vi "Init UAV Marker Position.vi"(0 "GMAP Control ref":refnum<k24>, 5 "Overlay Ref":refnum<k24>, 7 "lat":dbl=-31.1105459 format="%#_13g", 9 "lng":dbl=150.8617687 format="%#_13g", 11 "error in (no error)":errorcluster) -> (15 "error out":errorcluster)   [LabVIEW 2014]
uses:
  C:/Robotic Systems/Products/AgFalcon/Software/Ground Station/Data/Mapping DLL/GMap.NET.WindowsForms.dll
  Data/Mapping DLL/GMap.NET.WindowsForms.dll
  Aircraft Information/Controls/Aircraft GPS Data.ctl
  Aircraft Information/Controls/GPS Fix Type.ctl
  System.Drawing
  C:/Robotic Systems/Products/AgFalcon/Software/Ground Station/Data/Mapping DLL/GMap.NET.Core.dll
  Data/Mapping DLL/GMap.NET.Core.dll
  Aircraft Information/Sub VI/Set Aircraft GPS.vi
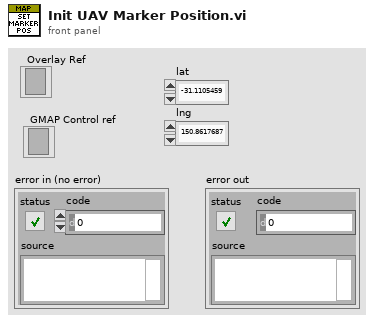
[diagram p1: front panel]
types:
  T1 = typedef "Aircraft GPS Data.ctl" = cluster{"Latitude (degrees)":dbl, "Longitude (degrees)":dbl, "Altitude (m)":dbl, "Fix Type":T2, "HDOP (cm)":u16, "VDOP (cm)":u16, "Ground Speed (m/s)":dbl, "Coarse Over Ground (degrees)":u16, "Number of Satellites":u8}
  T2 = typedef "GPS Fix Type.ctl" = enum16{"No Fix 0", "No Fix 1", "2D Fix", "3D Fix", "DGPS", "RTK"}
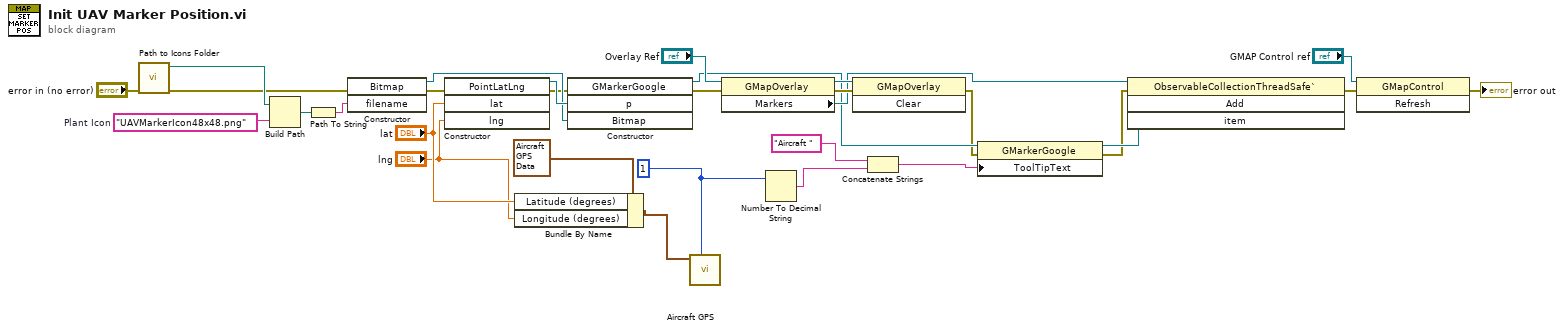
[diagram p0: block diagram]
diagram:
  w2 = u8 1 ("Aircraft ID")
  w18 = "UAVMarkerIcon48x48.png"  # Plant Icon
  n1 = call "Path to Icons Folder.vi"("Error In"="error in (no error)") -> ("Error Out"=w15:errorcluster, "Path to Icons Folder"=w19:path)  [unwired: 9 in]
  n2 = Build Path(base path=w19, name or relative path=w18) -> (appended path=w17:path)
  n3 = Path To String(path=w17) -> (string=w28:string)
  n4 = constructor class="Bitmap"(error in=w15, "filename"=w28) -> (reference out=w21:refnum<k24>, error out=w14:errorcluster)  [unwired: 2 in, 2 out]
  n5 = constructor class="PointLatLng"(error in=w14, "lat"="lat", "lng"="lng") -> (reference out=w27:refnum<k24>, error out=w13:errorcluster)  [unwired: 2 in, 3 out]
  n6 = Bundle By Name(cluster=T1 {"Latitude (degrees)"=0.0, "Longitude (degrees)"=0.0, "Altitude (m)"=0.0, "Fix Type"=enum."No Fix 0", "HDOP (cm)"=0, "VDOP (cm)"=0, "Ground Speed (m/s)"=0.0, "Coarse Over Ground (degrees)"=0, "Number of Satellites"=0} ("Aircraft Att Data Out"), "Latitude (degrees)"="lat", "Longitude (degrees)"="lng") -> (w1:T1)
  n7 = constructor class="GMarkerGoogle"(error in=w13, "p"=w27, "Bitmap"=w21) -> (reference out=w9:refnum<k24>, error out=w30:errorcluster)  [unwired: 2 in, 3 out]
  n8 = call-poly "Aircraft GPS.vi"("Aircraft ID"=w2, "Aircraft Att Data IN"=w1) -> ()  [unwired: 8 in, 2 out]
  n9 = property class="GMapOverlay"(reference="Overlay Ref", error in=w30) -> (reference out=w23:refnum<k24>, error out=w22:errorcluster, "Markers"=w20:refnum<k24>)
  n10 = Number To Decimal String(number=w2) -> (decimal integer string=w5:string)  [unwired: 1 in]
  n11 = invoke class="GMapOverlay" method="Clear"(reference=w23, error in=w22) -> (error out=w8:errorcluster)  [unwired: 1 in, 2 out]
  n12 = Concatenate Strings("Aircraft " ("string"), w5) -> (w3:string)
  n13 = property class="GMarkerGoogle"(reference=w9, error in=w8, "ToolTipText"=w3) -> (reference out=w7:refnum<k24>, error out=w6:errorcluster)
  n14 = invoke class="ObservableCollectionThreadSafe`" method="Add"(reference=w20, error in=w6, "item"=w7) -> (error out=w29:errorcluster)  [unwired: 1 in, 3 out]
  n15 = invoke class="GMapControl" method="Refresh"(reference="GMAP Control ref", error in=w29) -> (error out=→"error out":errorcluster)  [unwired: 1 in, 2 out]
